vi "LVClass_CorrectionDataManager ctor from InteractionMatrixFile.vi"(0 "CorrectionDataManager (const)":refnum<class "CorrectionDataManager.lvclass">, 5 "Haso config file path":path, 7 "Interaction matrix path":path, 11 "error in (no error)":errorcluster) -> (4 "CorrectionDataManager (new)":refnum<class "CorrectionDataManager.lvclass">, 15 "error out":errorcluster)   [LabVIEW 2020, in "CorrectionDataManager.lvclass"]
doc: "CorrDataManager constructor from a CorrDataManager dump file.\n\n<B>corrdata_managerIn</B> : Constant Pointer to CorrDataManager object.\n<B>corrdata_managerOut</B> : Constant Pointer to CorrDataManager object.\n<B>haso_config_file_path</B> : Absolute path to Haso configuration file.\n<B>interaction_matrix_file_path</B> : Absolute path to CorrDataManager dump file.\n<B>use_phase</B> : use phase or slopes in correction process."
uses:
  CorrectionDataManager.lvclass
  Handle creation.ctl
  CorrectionDataManager.lvclass/CorrectionDataManager.ctl
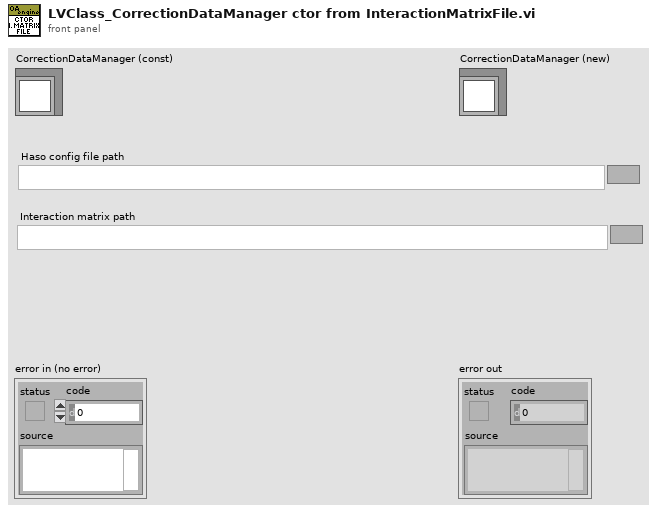
[diagram p1: front panel]
types:
  T1 = typedef "Handle creation.ctl" = enum16{"By ctor", "By write function"}
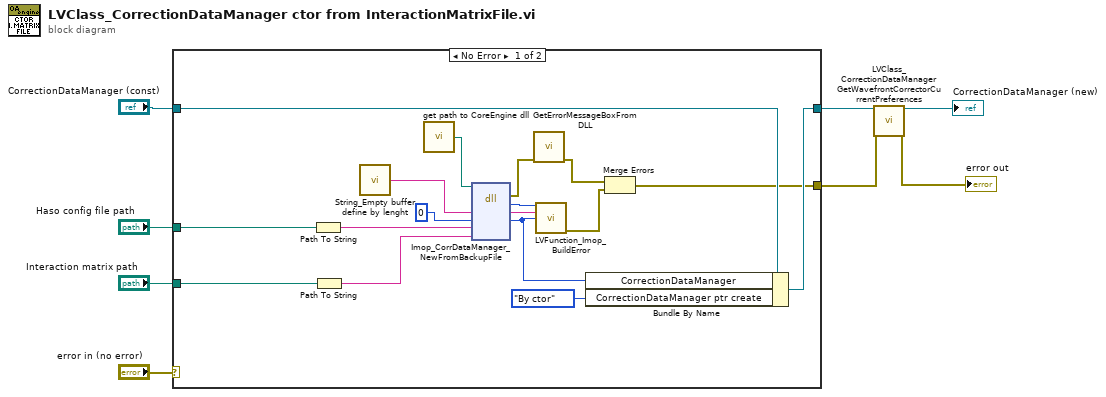
[diagram p0: block diagram]
diagram:
  n1 = case shown="No Error" "error in (no error)" {
    selector: "error in (no error)" -> [_ w27]
    tunnel: [w14 w27] -> w2
    tunnel: [w17 w26] -> w4
    tunnel: "CorrectionDataManager (const)" -> [w18 w26]
    tunnel: "Interaction matrix path" -> [w13 _]
    tunnel: "Haso config file path" -> [w11 _]
    frame No Error {
      n2 = Path To String(path=w11) -> (string=w10:string)
      n3 = Path To String(path=w13) -> (string=w12:string)
      n4 = call "String_Empty buffer define by lenght.vi"() -> ("Empty buffer"=w25:string)  [unwired: 1 in]
      n5 = call "get path to CoreEngine dll.vi"() -> ("path to wavekit library"=w22:path)  [unwired: 14 in, 1 out]
      n6 = dll-call lib="D:/soft/HASO_v3/SVN_trunk/ImOpCoreEngine4_LV2011/DLLs/c_interface_vc100.dll" fn="Imop_CorrDataManager_NewFromBackupFile"(path in=w22, "message"=w25, "WavefrontCorrection"=0 ("Pupil"), "haso_config_file_path"=w10, "Interaction matrix path"=w12) -> (error out=w21:errorcluster, "return type"=w23:i32, "message"=w24:string, "WavefrontCorrection"=w9:i64)  [unwired: 4 in, 1 out]
      n7 = call "GetErrorMessageBoxFromDLL.vi"("error IN"=w21) -> ("error OUT"=w16:errorcluster)  [unwired: 10 in]
      n8 = call "LVFunction_Imop_BuildError.vi"("code"=w23, "String to Prepend to source (\"\")"=w24, "Adresse"=w9) -> ("error out"=w15:errorcluster)  [unwired: 12 in]
      n9 = Bundle By Name(cluster=w18, "CorrectionDataManager"=w9, "CorrectionDataManager ptr create"=Handle_creation."By ctor" ("Pupil ptr create")) -> (w17:refnum<class "CorrectionDataManager.lvclass">)
      n10 = Merge Errors(w16, w15) -> (w14:errorcluster)
    }
    frame Error {
    }
  }
  n11 = call "LVClass_CorrectionDataManager GetWavefrontCorrectorCurrentPreferences.vi"("CorrectionDataManager in"=w4, "error in (no error)"=w2) -> ("CorrectionDataManager out"=→"CorrectionDataManager (new)":refnum<class "CorrectionDataManager.lvclass">, "error out"=→"error out":errorcluster)  [unwired: 11 in, 1 out]
